vi "Get Session and Channel (1 Pin).vi"(8 "error in (no error)":errorcluster, 9 "site (-1)":i32=-1, 10 "pin name":string, 11 "session information":T1[](array[typedef])) -> (0 "error out":errorcluster, 2 "channel list":string[](array[string]), 3 "session index":i32)   [LabVIEW 2020, in "Measurement Service Helpers.lvlib"]
doc: "Gets the session index and channel list for the session that corresponds to the given pin name input. The session index can be used to access the given session information array.\nThis VI only returns a single matching session and produces an error if multiple sessions match the criteria."
uses:
  Measurement Service Helpers.lvlib
  <vilib>/MeasurementLink/MeasurementLink Session Management Client/RPC Messages/ni_measurementlink_sessionmanagement_v1_ChannelMapping.ctl
  <vilib>/MeasurementLink/MeasurementLink Session Management Client/MeasurementLink Session Management Client.lvlib
  <vilib>/MeasurementLink/MeasurementLink Session Management Client/RPC Messages/nidevice_grpc_Session.ctl
  <vilib>/MeasurementLink/MeasurementLink Session Management Client/RPC Messages/ni_measurementlink_sessionmanagement_v1_SessionInformation.ctl
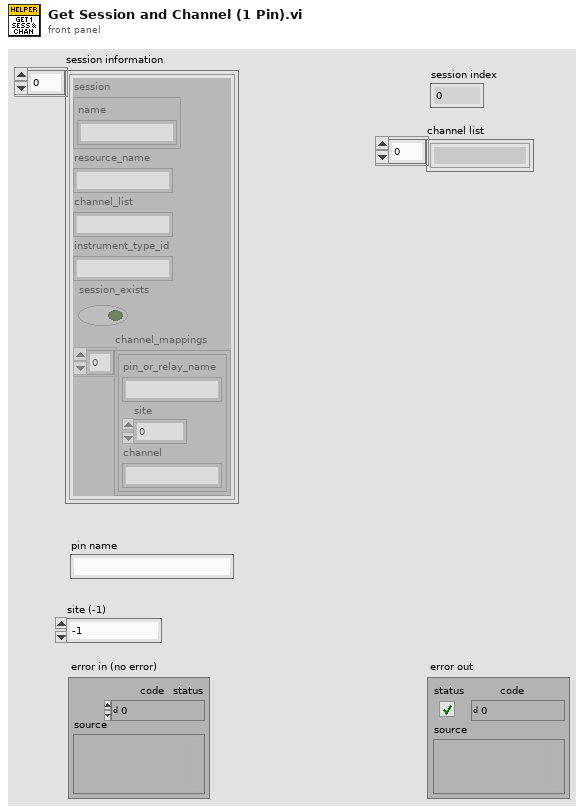
[diagram p1: front panel]
types:
  T1 = typedef "MeasurementLink Session Management Client.lvlib/ni_measurementlink_sessionmanagement_v1_SessionInformation.ctl" = cluster{"session":T2, "resource_name":string, "channel_list":string, "instrument_type_id":string, "session_exists":bool, "channel_mappings":T3[]}
  T2 = typedef "MeasurementLink Session Management Client.lvlib/nidevice_grpc_Session.ctl" = cluster{"name":string}
  T3 = typedef "MeasurementLink Session Management Client.lvlib/ni_measurementlink_sessionmanagement_v1_ChannelMapping.ctl" = cluster{"pin_or_relay_name":string, "site":i32, "channel":string}
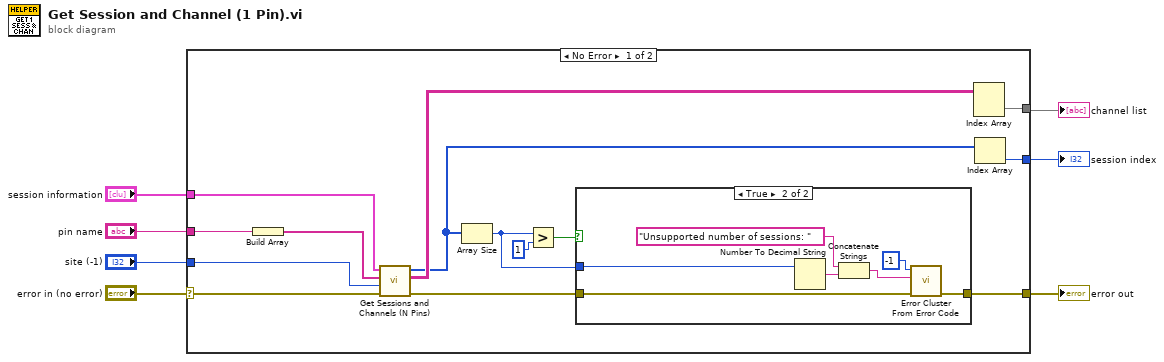
[diagram p0: block diagram]
diagram:
  n1 = case shown="No Error" "error in (no error)" {
    selector: "error in (no error)" -> [w21 w30]
    tunnel: [w20 w30] -> w6
    tunnel: "session information" -> [w18 _]
    tunnel: "pin name" -> [w17 _]
    tunnel: "site (-1)" -> [w15 _]
    tunnel: [w12 _] -> w2
    tunnel: [w10 _] -> w1
    frame No Error {
      n2 = Build Array(w17) -> (w16:string[])
      n3 = call "Get Sessions and Channels (N Pins).vi"("error in (no error)"=w21, "site (-1)"=w15, "pin names"=w16, "session information"=w18) -> ("error out"=w19:errorcluster, "channel list"=w11:string[][], "session indexes"=w9:i32[])  [unwired: 5 in]
      n4 = Array Size(array=w9) -> (size(s)=w8:i32)
      n5 = Greater?(x=w8, y=1) -> (0:w13:bool)
      n6 = case shown="True" w13 {
        tunnel: w19 -> [w22 w25]
        tunnel: [w22 w24] -> w20
        tunnel: w8 -> [_ w23]
        frame False {
        }
        frame True {
          n7 = Number To Decimal String(number=w23) -> (decimal integer string=w27:string)  [unwired: 1 in]
          n8 = Concatenate Strings("Unsupported number of sessions: " ("error message (\"\")"), w27) -> (w26:string)
          n9 = call <vilib>:"Error Cluster From Error Code.vi"("error in (no error)"=w25, "error message (\"\")"=w26, "error code (0)"=-1) -> ("error out"=w24:errorcluster)  [unwired: 6 in]
        }
      }
      n10 = Index Array(array=w11) -> (element=w12:string[])  [unwired: 2 in]
      n11 = Index Array(array=w9) -> (element=w10:i32)  [unwired: 1 in]
    }
    frame Error {
    }
  }
  "error out" <- w6
  "channel list" <- w2
  "session index" <- w1
